vi "Create Event.vi"(6 "end":timestamp format="%<%X\n%x>T", 7 "start":timestamp format="%<%X\n%x>T", 8 "error in (no error)":errorcluster, 9 "title":string, 10 "database item id":u32, 11 "eLab in":refnum<class "PL eLabFTW Client.lvclass">) -> (0 "error out":errorcluster, 2 "event id":u32, 3 "eLab out":refnum<class "PL eLabFTW Client.lvclass">)   [LabVIEW 2015, in "PL eLabFTW Client.lvclass"]
doc: "Creates new event and returns new event id."
uses:
  PL eLabFTW Client.lvclass
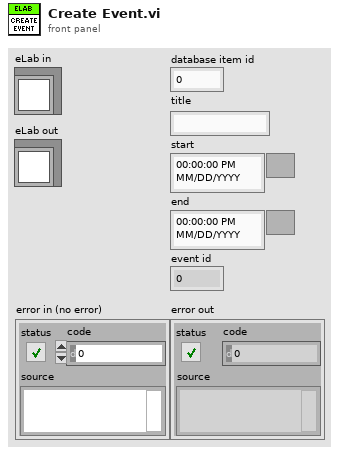
[diagram p1: front panel]
types:
  T1 = cluster{"format string":string, "title":string}[]
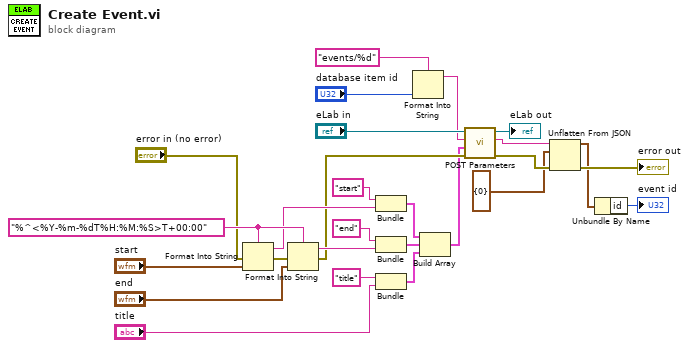
[diagram p0: block diagram]
diagram:
  w17 = "%^<%Y-%m-%dT%H:%M:%S>T+00:00" ("format string")
  n1 = Format Into String(format string=w17, error in="error in (no error)", "start") -> (resulting string=w14:string, error out=w18:errorcluster)  [unwired: 1 in]
  n2 = Format Into String(format string=w17, error in=w18, "end") -> (resulting string=w13:string, error out=w5:errorcluster)  [unwired: 1 in]
  n3 = Bundle("format string"="start", w14) -> (w8:cluster{"format string":string, string})  [unwired: 1 in]
  n4 = Bundle("format string"="end", w13) -> (w9:cluster{"format string":string, string})  [unwired: 1 in]
  n5 = Bundle("format string"="title", "title"="title") -> (w7:cluster{"format string":string, "title":string})  [unwired: 1 in]
  n6 = Format Into String(format string="events/%d", "database item id") -> (resulting string=w1:string)  [unwired: 2 in, 1 out]
  n7 = Build Array(w8, w9, w7) -> (w4:T1)
  n8 = call "POST Parameters.vi"("error in (no error)"=w5, "parameters"=w4, "relative URL"=w1, "eLab in"="eLab in") -> ("error out"=w25:errorcluster, "response body"=w21:string, "eLab out"=→"eLab out":refnum<class "PL eLabFTW Client.lvclass">)  [unwired: 5 in]
  n9 = Unflatten From JSON(JSON string=w21, type and defaults=cluster{"id":u32} {"id"=0}, error in (no error)=w25) -> (value=w22:cluster{"id":u32}, error out=→"error out":errorcluster)  [unwired: 4 in]
  n10 = Unbundle By Name(w22) -> ("id"=→"event id":u32)
